vi "Plain Text.vi"(7 "Strip End? (F)":bool, 8 "error in (no error)":errorcluster, 11 "TermLine in":refnum<class "TermLine.lvclass">) -> (0 "error out":errorcluster, 2 "Line":string, 3 "TermLine out":refnum<class "TermLine.lvclass">)   [LabVIEW 2020, in "Terminal.lvlib" / "TermLine.lvclass"]
uses:
  TermLine.lvclass
  <vilib>/Utility/error.llb/whitespace.ctl
  TermLine.lvclass/TermLine.ctl
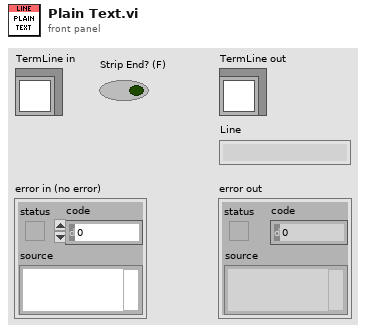
[diagram p1: front panel]
types:
  T1 = typedef "Terminal.lvlib/TermLine.lvclass/Ref Data.ctl" = cluster{"Chars":T2[], "Width":i32}
  T2 = typedef "Terminal.lvlib/Term Char.ctl" = cluster{"Char":string, "FG":u32, "BG":u32}
  T3 = typedef "whitespace.ctl" = u16
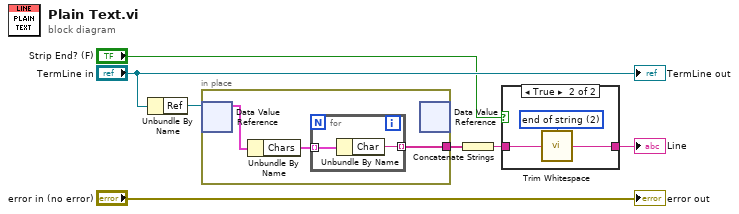
[diagram p0: block diagram]
diagram:
  n1 = Unbundle By Name("TermLine in") -> ("Ref"=w6:refnum<data-value>)
  n2 = in-place {
    in-place-border: [w8] -> w4
    n3 = in-place-dvr #1(w6) -> (w10:T1)  [unwired: 1 out]
    n4 = Unbundle By Name(w10) -> ("Chars"=w9:T2[])
    n5 = for {
      tunnel: w9 -> [w12] mode=indexing
      tunnel: [w11] -> w8 mode=indexing
      n6 = Unbundle By Name(w12) -> ("Char"=w11:string)
    }
    n7 = in-place-dvr #1() -> ()  [unwired: 1 in, 2 out]
  }
  n8 = Concatenate Strings(w4) -> (w3:string)
  n9 = case shown="True" "Strip End? (F)" {
    tunnel: w3 -> [w13 w16]
    tunnel: [w13 w14] -> w2
    frame False {
    }
    frame True {
      w15 = T3 2 items=["both", "start of string", "end of string"] ("location (both)")
      n10 = call <vilib>:"Trim Whitespace.vi"("string"=w16, "location (both)"=w15) -> ("trimmed string"=w14:string)
    }
  }
  "Line" <- w2
  "error out" <- "error in (no error)"
  "TermLine out" <- "TermLine in"
